vi "Update GUI.vi"(8 "error in (no error)":errorcluster, 11 "Microscope Controller in":refnum<class "Microscope Controller.lvclass">) -> (0 "error out":errorcluster, 3 "Microscope Controller out":refnum<class "Microscope Controller.lvclass">)   [LabVIEW 2020, in "Microscope.lvlib" / "Microscope Controller.lvlib" / "Microscope Controller.lvclass"]
uses:
  Microscope Controller.lvclass
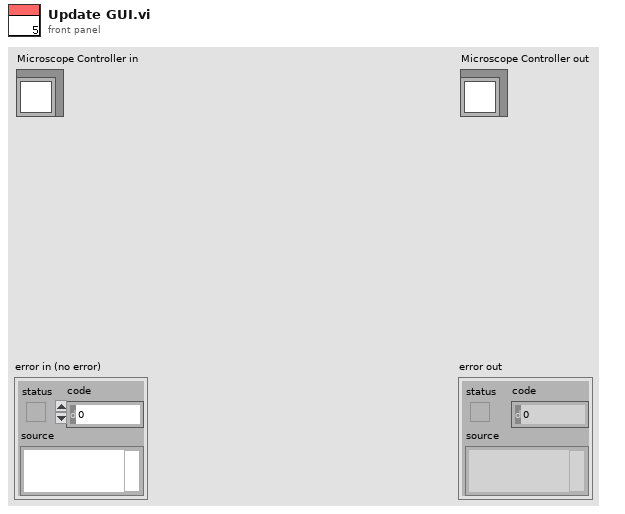
[diagram p1: front panel]
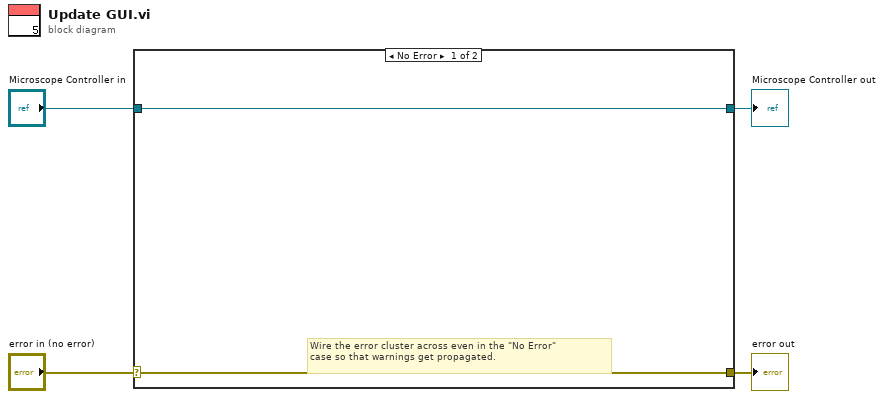
[diagram p0: block diagram]
diagram:
  n1 = case shown="No Error" "error in (no error)" {
    selector: "error in (no error)" -> [w5 w8]
    tunnel: [w5 w8] -> w3
    tunnel: [w6 w7] -> w1
    tunnel: "Microscope Controller in" -> [w6 w7]
    frame No Error {
      # "Wire the error cluster across even in the \"No Error\"\ncase so that warnings get propagated."
    }
    frame Error {
    }
  }
  "error out" <- w3
  "Microscope Controller out" <- w1
